vi "Append Fail Result.vi"(7 "Description":string, 8 "error in (no error)":errorcluster, 9 "Message":string, 10 "Result Type":T1, 11 "LUnit Test Case In":refnum<class "LUnit Inheriting Test Case.lvclass">) -> (0 "error out":errorcluster, 3 "LUnit Test Case Out":refnum<class "LUnit Inheriting Test Case.lvclass">)   [LabVIEW 2020]
doc: "Generates a fail result for the calling test method. A description and message may be provided."
uses:
  Core/Result/Status.ctl
  Core/Result/Result.lvlib
  Core/Result/Type.ctl
  Core/Result/Result.ctl
  LUnit Inheriting Test Case.lvclass
  C:/git/astemes-lunit/source/API/LUnit Test Case/LUnit Test Case.lvclass
  C:/git/astemes-lunit/source/Core/Runnable/Runnable.lvclass
  C:/git/astemes-lunit/source/API/LUnit Inheriting Test Case/LUnit Test Case/LUnit Inheriting Test Case.lvclass
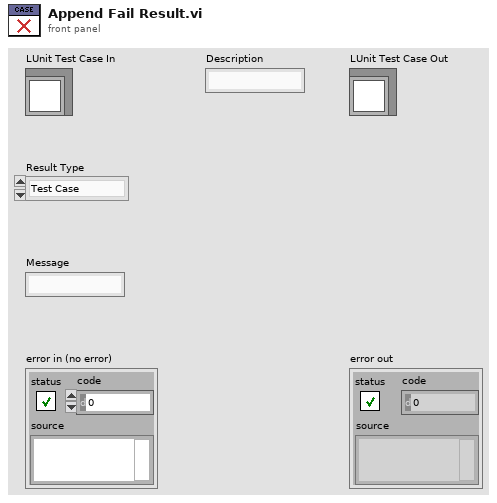
[diagram p1: front panel]
types:
  T1 = typedef "Result.lvlib/Type.ctl" = enum16{"Test Case", "Test Suite", "Test Run", "Pass", "Fail", "Skip", "Pass if", "Fail if", "Pass if Error", "Fail if Error", "Pass if Equal", "Fail if Equal"}
  T2 = typedef "Result.lvlib/Status.ctl" = enum16{"", "Passed", "Failed", "Error", "Skipped", "Setup Error", "Broken", "Teardown Error"}
  T3 = typedef "Result.lvlib/Result.ctl" = cluster{"Name":string, "Message":string, "Description":string, "Status":T2, "Result Type":T1, "Execution Time":dbl}
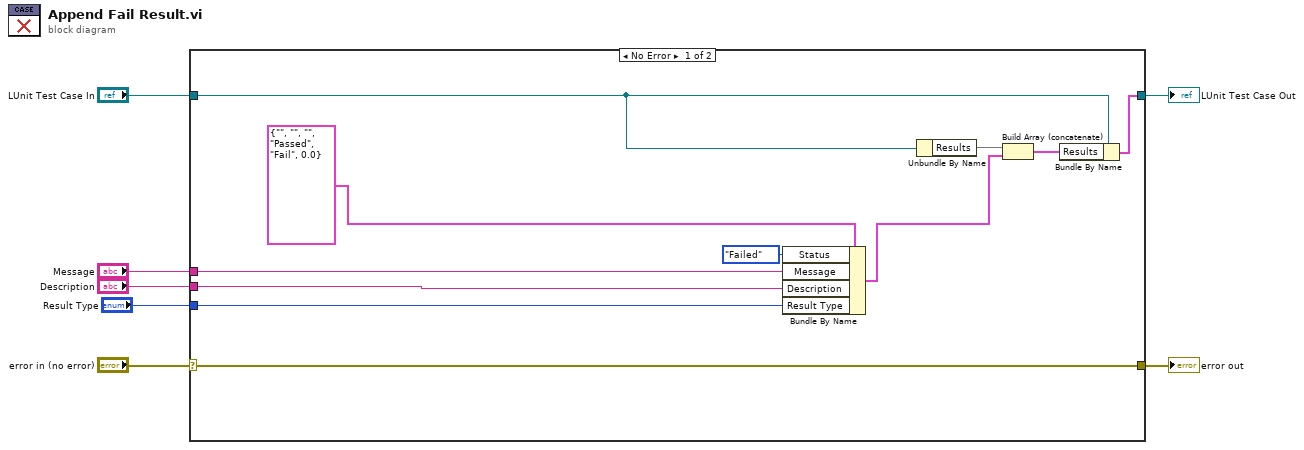
[diagram p0: block diagram]
diagram:
  n1 = case shown="No Error" "error in (no error)" {
    selector: "error in (no error)" -> [w16 w19]
    tunnel: "Message" -> [w18 _]
    tunnel: "Description" -> [w17 _]
    tunnel: [w16 w19] -> w4
    tunnel: [w14 w20] -> w3
    tunnel: "LUnit Test Case In" -> [w13 w20]
    tunnel: "Result Type" -> [w11 _]
    frame No Error {
      n2 = Bundle By Name(cluster=T3 {"Name"="", "Message"="", "Description"="", "Status"=enum."Passed", "Result Type"=enum."Fail", "Execution Time"=0.0} ("Temporary Assertion Result"), "Status"=Status."Failed", "Message"=w18, "Description"=w17, "Result Type"=w11) -> (w12:T3)
      n3 = Unbundle By Name(w13) -> ("Results"=w10)
      n4 = Build Array (concatenate)(w10, w12) -> (w9:T3[])
      n5 = Bundle By Name(cluster=w13, "Results"=w9) -> (w14:cluster{})
    }
    frame Error {
    }
  }
  "error out" <- w4
  "LUnit Test Case Out" <- w3
